vi "read default menu name.vi"(8 "error in":errorcluster, 11 "module editor node in":refnum<class "module editor node.lvclass">) -> (0 "error out":errorcluster, 2 "default menu name":string, 3 "module editor node out":refnum<class "module editor node.lvclass">)   [LabVIEW 2013]
uses:
  module editor node.lvclass
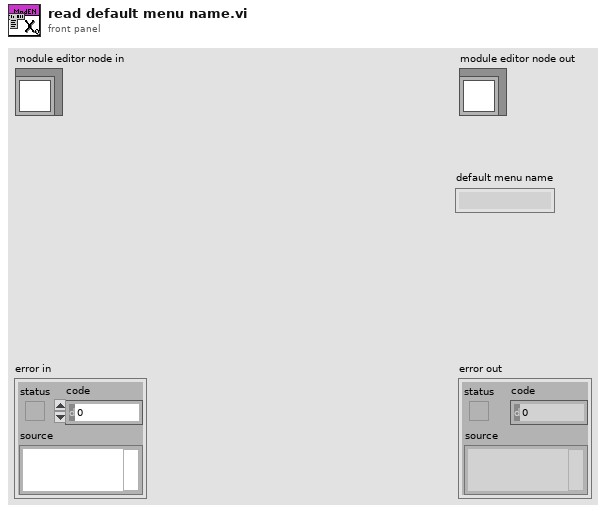
[diagram p1: front panel]
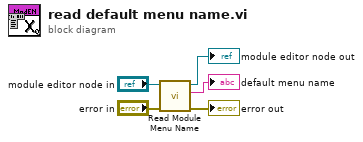
[diagram p0: block diagram]
diagram:
  n1 = call-dynamic "Read Module Menu Name.vi"("error in"="error in", "module editor node in"="module editor node in") -> ("error out"=→"error out":errorcluster, "menu name"=→"default menu name":string, "module editor node out"=→"module editor node out":refnum<class "module editor node.lvclass">)  [unwired: 7 in]
